vi "SMD7615 UDP Stop Move.vi"(8 "error in (no error)":errorcluster, 10 "IP":string="192.168.1.30", 11 "connection ID in":refnum<k16>) -> (0 "error out":errorcluster, 3 "connection ID out":refnum<k16>)   [LabVIEW 2016, in "SMD-7615.lvlib" / "eSCL.lvlib"]
uses:
  eSCL.lvlib
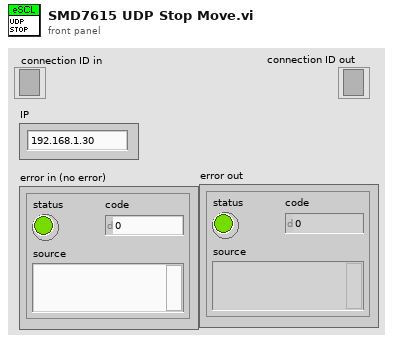
[diagram p1: front panel]
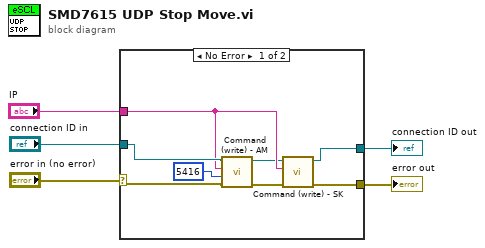
[diagram p0: block diagram]
diagram:
  n1 = case shown="No Error" "error in (no error)" {
    selector: "error in (no error)" -> [w12 w14]
    tunnel: "connection ID in" -> [w13 w15]
    tunnel: [w7 w15] -> w3
    tunnel: [w9 w14] -> w2
    tunnel: "IP" -> [w8 _]
    frame No Error {
      n2 = call "Command (write) - AM.vi"("error in (no error)"=w12, "Max. Acceleration"=5416 ("Acceleration"), "IP"=w8, "connection ID in"=w13) -> ("error out"=w10:errorcluster, "connection ID out"=w6:refnum<k16>)  [unwired: 6 in]
      n3 = call "Command (write) - SK.vi"("error in (no error)"=w10, "IP"=w8, "connection ID in"=w6) -> ("error out"=w9:errorcluster, "connection ID out"=w7:refnum<k16>)  [unwired: 7 in]
    }
    frame Error {
    }
  }
  "connection ID out" <- w3
  "error out" <- w2
